vi "trace manipulation.vi"() -> ()   [LabVIEW 2016]
panel:
  out "Output array":dbl[](array[numeric])
  out "Waveform Graph":dbl[](graph)
  out "Linear frequecny increment":dbl format="%#_13g"
  out "Stop frequency(MHz)":dbl format="%#_13g"
  out "Start frequency (MHz)":dbl format="%#_13g"
  out "VISA resource out":refnum<visa-resource-name>
  out "Number of points":i32
  out "Trace Array (1D)":dbl[](array[numeric])
  in  "Trace":enum16{"Trace1", "Trace2", "Trace3"}(ring)
  in  "VISA resource name":refnum<visa-resource-name>
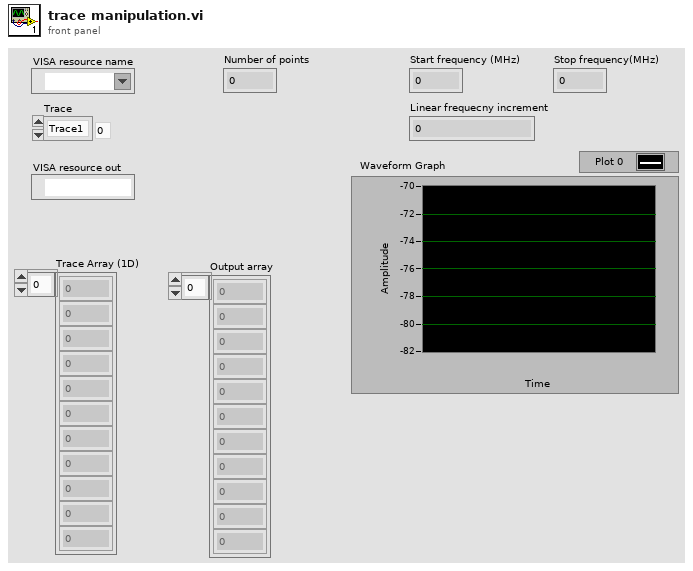
[diagram p1: front panel]
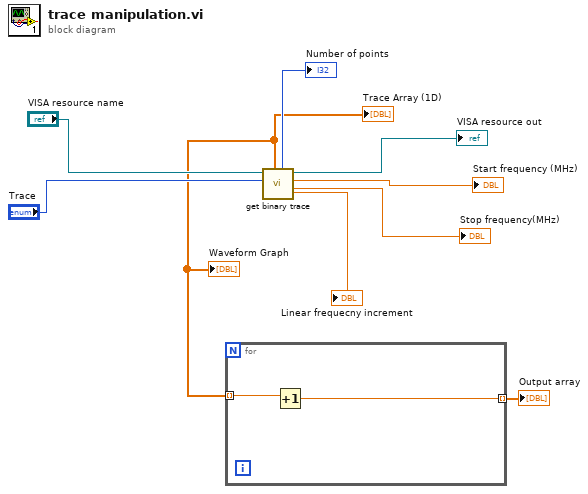
[diagram p0: block diagram]
diagram:
  n1 = call "get binary trace.vi"("Trace Name (0:Trace1)"="Trace", "VISA resource in"="VISA resource name") -> ("Stop frequency(MHz)"=→"Stop frequency(MHz)":dbl, "Start frequency (MHz)"=→"Start frequency (MHz)":dbl, "VISA resource out"=→"VISA resource out":refnum<visa-resource-name>, "Number of points"=→"Number of points":i32, "Linear frequecny increment"=→"Linear frequecny increment":dbl, "Trace Array (1D)"=w2:dbl[])  [unwired: 2 in, 1 out]
  "Trace Array (1D)" <- w2
  "Waveform Graph" <- w2
  n2 = for {
    tunnel: w2 -> [w11] mode=indexing
    tunnel: [w10] -> w1 mode=indexing
    n3 = Increment(x=w11) -> (x+1=w10:dbl)
  }
  "Output array" <- w1
